vi "Output Digital Code.vi"(4 "V- (Not Working":dbl, 5 "V+ (Not Working)":dbl=4.5, 6 "error in (no error)":errorcluster, 8 "Pulse Time":dbl=0.01 min=0.0 step=1e-09 format="%#.3f", 9 "Input":i8 min=0 step=1 format="%#.3f") -> (0 "error out":errorcluster)   [LabVIEW 2012]
uses:
  <vilib>/DAQmx/write.llb/DAQmx Write (Digital Bool 1Line 1Point).vi
  <vilib>/DAQmx/create/channels.llb/DAQmx Create Channel (DO-Digital Output).vi
  <vilib>/DAQmx/miscellaneous.llb/DAQmx Fill In Error Info.vi
panel:
  out "Pin 7":bool
  out "Pin 6":bool
  out "Pin 5":bool
  out "Pin 4":bool
  out "Pin 3":bool
  out "Pin 2":bool
  out "Pin 1":bool
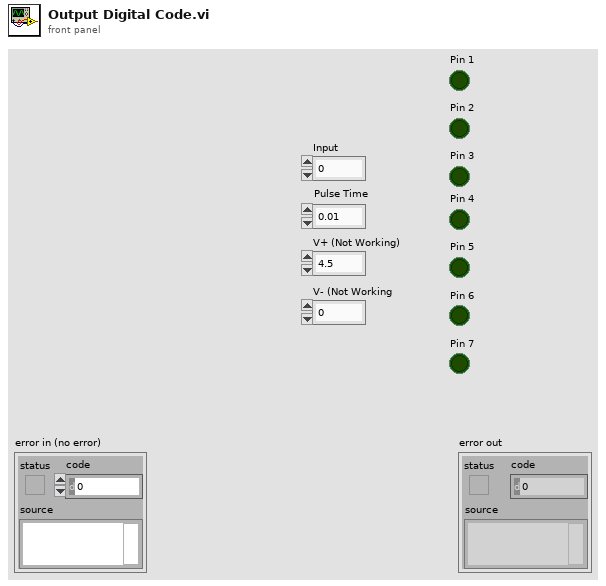
[diagram p1: front panel]
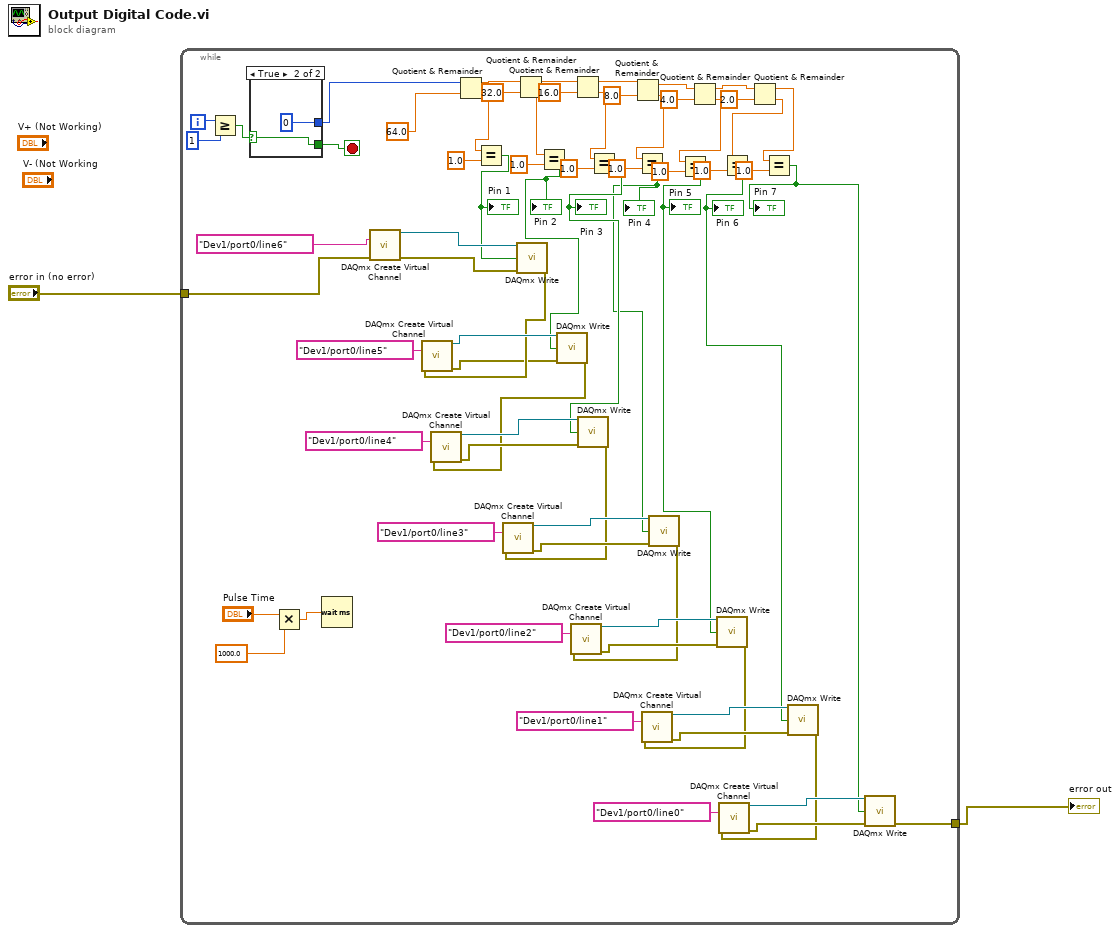
[diagram p0: block diagram]
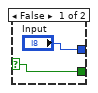
[diagram p2: hidden frame]
diagram:
  n1 = while {
    tunnel: "error in (no error)" -> [w25]
    tunnel: [w11] -> w1
    i -> [w10]
    stop <- w9 stop-if-true
    n2 = Greater Or Equal?(x=w10, y=1) -> (x >= y?=w7:bool)
    n3 = case shown="True" w7 {
      selector: w7 -> [w72 w74]
      tunnel: [w72 w74] -> w9
      tunnel: ["Input" 0] -> w6
      frame False {
      }
      frame True {
      }
    }
    n4 = Multiply(x="Pulse Time", y=1000.0) -> (x*y=w3:dbl)
    n5 = Wait (ms)(milliseconds to wait=w3) -> ()  [unwired: 1 out]
    n6 = call-poly <vilib>:"DAQmx Create Virtual Channel.vi"("lines"=tag "Dev1/port0/line6", "error in"=w25) -> ("task out"=w46:refnum<k21>, "error out"=w24:errorcluster)  [unwired: 4 in, 8 out]
    n7 = Quotient & Remainder(x=w6, y=64.0) -> (x-y*floor(x/y)=w70:dbl, floor(x/y)=w55:dbl)
    n8 = Equal?(x=w55, y=1.0) -> (x = y?=w40:bool)
    "Pin 1" <- w40
    n9 = Quotient & Remainder(x=w70, y=32.0) -> (x-y*floor(x/y)=w69:dbl, floor(x/y)=w54:dbl)
    n10 = call-poly <vilib>:"DAQmx Write.vi"("task/channels in"=w46, "data"=w40, "error in"=w24) -> ("error out"=w23:errorcluster)  [unwired: 1 in, 11 out]
    n11 = call-poly <vilib>:"DAQmx Create Virtual Channel.vi"("lines"=tag "Dev1/port0/line5", "error in"=w23) -> ("task out"=w43:refnum<k21>, "error out"=w22:errorcluster)  [unwired: 4 in, 8 out]
    n12 = Equal?(x=w54, y=1.0) -> (x = y?=w39:bool)
    "Pin 2" <- w39
    n13 = call-poly <vilib>:"DAQmx Write.vi"("task/channels in"=w43, "data"=w39, "error in"=w22) -> ("error out"=w16:errorcluster)  [unwired: 1 in, 11 out]
    n14 = call-poly <vilib>:"DAQmx Create Virtual Channel.vi"("lines"=tag "Dev1/port0/line4", "error in"=w16) -> ("task out"=w42:refnum<k21>, "error out"=w21:errorcluster)  [unwired: 4 in, 8 out]
    n15 = Quotient & Remainder(x=w69, y=16.0) -> (x-y*floor(x/y)=w68:dbl, floor(x/y)=w53:dbl)
    n16 = Equal?(x=w53, y=1.0) -> (x = y?=w38:bool)
    "Pin 3" <- w38
    n17 = call-poly <vilib>:"DAQmx Write.vi"("task/channels in"=w42, "data"=w38, "error in"=w21) -> ("error out"=w15:errorcluster)  [unwired: 1 in, 11 out]
    n18 = call-poly <vilib>:"DAQmx Create Virtual Channel.vi"("lines"=tag "Dev1/port0/line3", "error in"=w15) -> ("task out"=w37:refnum<k21>, "error out"=w20:errorcluster)  [unwired: 4 in, 8 out]
    n19 = Quotient & Remainder(x=w68, y=8.0) -> (x-y*floor(x/y)=w49:dbl, floor(x/y)=w52:dbl)
    n20 = Equal?(x=w52, y=1.0) -> (x = y?=w29:bool)
    "Pin 4" <- w29
    n21 = call-poly <vilib>:"DAQmx Write.vi"("task/channels in"=w37, "data"=w29, "error in"=w20) -> ("error out"=w14:errorcluster)  [unwired: 1 in, 11 out]
    n22 = call-poly <vilib>:"DAQmx Create Virtual Channel.vi"("lines"=tag "Dev1/port0/line2", "error in"=w14) -> ("task out"=w35:refnum<k21>, "error out"=w19:errorcluster)  [unwired: 4 in, 8 out]
    n23 = Quotient & Remainder(x=w49, y=4.0) -> (x-y*floor(x/y)=w48:dbl, floor(x/y)=w51:dbl)
    n24 = Equal?(x=w51, y=1.0) -> (x = y?=w28:bool)
    "Pin 5" <- w28
    n25 = call-poly <vilib>:"DAQmx Write.vi"("task/channels in"=w35, "data"=w28, "error in"=w19) -> ("error out"=w13:errorcluster)  [unwired: 1 in, 11 out]
    n26 = call-poly <vilib>:"DAQmx Create Virtual Channel.vi"("lines"=tag "Dev1/port0/line1", "error in"=w13) -> ("task out"=w33:refnum<k21>, "error out"=w18:errorcluster)  [unwired: 4 in, 8 out]
    n27 = Quotient & Remainder(x=w48, y=2.0) -> (x-y*floor(x/y)=w47:dbl, floor(x/y)=w50:dbl)
    n28 = Equal?(x=w50, y=1.0) -> (x = y?=w27:bool)
    "Pin 6" <- w27
    n29 = Equal?(x=w47, y=1.0) -> (x = y?=w26:bool)
    "Pin 7" <- w26
    n30 = call-poly <vilib>:"DAQmx Write.vi"("task/channels in"=w33, "data"=w27, "error in"=w18) -> ("error out"=w12:errorcluster)  [unwired: 1 in, 11 out]
    n31 = call-poly <vilib>:"DAQmx Create Virtual Channel.vi"("lines"=tag "Dev1/port0/line0", "error in"=w12) -> ("task out"=w31:refnum<k21>, "error out"=w17:errorcluster)  [unwired: 4 in, 8 out]
    n32 = call-poly <vilib>:"DAQmx Write.vi"("task/channels in"=w31, "data"=w26, "error in"=w17) -> ("error out"=w11:errorcluster)  [unwired: 1 in, 11 out]
  }
  "error out" <- w1
